vi "To Variant.vi"(0 "Obj in":refnum<class "Pulse Train.lvclass">, 11 "error in (no error)":errorcluster) -> (4 "Obj out":refnum<class "Pulse Train.lvclass">, 8 "Array":variant[](array[variant]), 15 "error out":errorcluster)   [LabVIEW 2020, in "Pulse Train.lvclass"]
uses:
  Pulse Train.lvclass
  Pulse Train.lvclass/Pulse Train.ctl
  Waveform/Waveform.lvclass
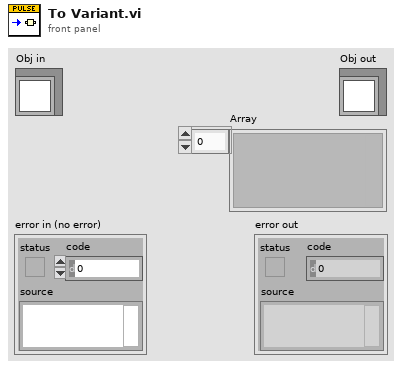
[diagram p1: front panel]
types:
  T1 = typedef "Pulse Train.lvclass/Serialized.ctl" = cluster{"Shape":string, "Width (us)":string, "Rate (Hz)":dbl}
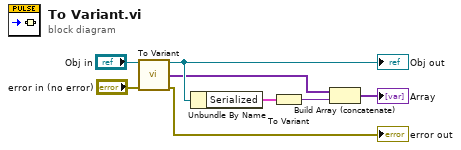
[diagram p0: block diagram]
diagram:
  n1 = call-parent "To Variant.vi"("Obj in"="Obj in", "error in (no error)"="error in (no error)") -> ("Obj out"=w3:refnum<class "Pulse Train.lvclass">, "Array"=w2:variant[], "error out"=→"error out":errorcluster)  [unwired: 11 in]
  "Obj out" <- w3
  n2 = Unbundle By Name(w3) -> ("Serialized"=w4:T1)
  n3 = To Variant(anything=w4) -> (Variant=w5:variant)
  n4 = Build Array (concatenate)(w2, w5) -> (→"Array":variant[])
